vi "Write File Refnum.vi"(10 "File Refnum":refnum<file>, 11 "Text File Sink in":refnum<class "Text File Sink.lvclass">) -> (3 "Text File Sink out":refnum<class "Text File Sink.lvclass">)   [LabVIEW 2016, in "Stream Log.lvlib" / "Text File Sink.lvclass"]
uses:
  <userlib>/Composed Systems/Stream/Log/Text File Sink/Text File Sink.lvclass
  <userlib>/Composed Systems/Stream/Log/Text File Sink/Text File Sink.lvclass/Text File Sink.ctl
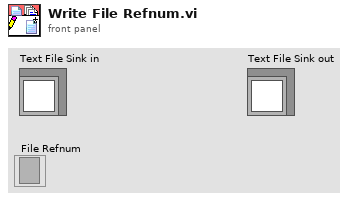
[diagram p1: front panel]
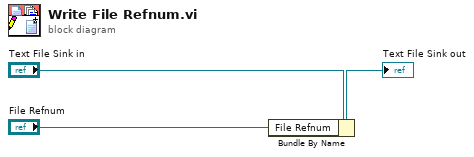
[diagram p0: block diagram]
diagram:
  n1 = Bundle By Name(cluster="Text File Sink in", "File Refnum"="File Refnum") -> (→"Text File Sink out":refnum<class "Text File Sink.lvclass">)
